vi "Read config file.vi"(3 "error in":errorcluster, 4 "file (use dialog)":path) -> (0 "error out":errorcluster, 1 "Drives":T2(array[cluster]))   [LabVIEW 2014]
uses:
  Axis enum.ctl
panel:
  out "Drive letters":string[](array[string])
  # "GUI=22\nAXES=2 CE\nC:XRT1=109\nE:XLA3=1250\nC:RANGE=360\nE:RANGE=50\nLEVEL=2\nCL=1"
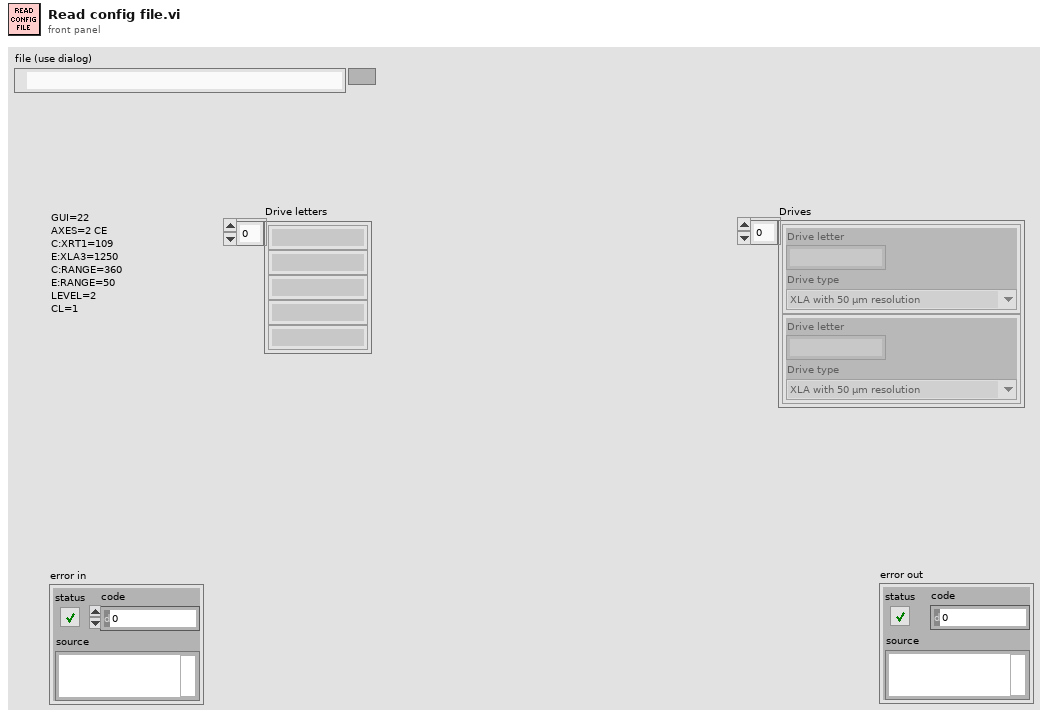
[diagram p1: front panel]
types:
  T1 = typedef "Axis enum.ctl" = enum16{"XLA with 50 µm resolution", "XLA with 10 µm resolution", "XLA with 1250 nm resolution", "XLA with 312 nm resolution", "XLA with 78 nm resolution", "XLS with 1250 nm resolution", "XLS with 312 nm resolution", "XLS with 78nm resolution", "XLS with 5nm resolution", "XLS with 1 nm resolution", "XRT-A with 109 µrad resolution", "XRT-U-30 with 109 µrad resolution", "XRT-U-30 with 49 µrad resolution", "XRT-U-30 with 19 µrad resolution", "XRT-U-30 with 3 µrad resolution", "XRT-U-40 with 109 µrad resolution", "XRT-U 40 with 49 µrad resolution", "XRT-U-40 with 19 µrad resolution", "XRT-U-40 with 3 µrad resolution", "XRT-U-60 with 109 µrad resolution", "XRT-U-60 with 49 µrad resolution", "XRT-U-60 with 19 µrad resolution", "XRT-U-60 with 3 µrad resolution"}
  T2 = cluster{"Drive letter":string, "Drive type":T1}[]
  T3 = cluster{"Name":string, "Data":string, "Enum type":T1}[]
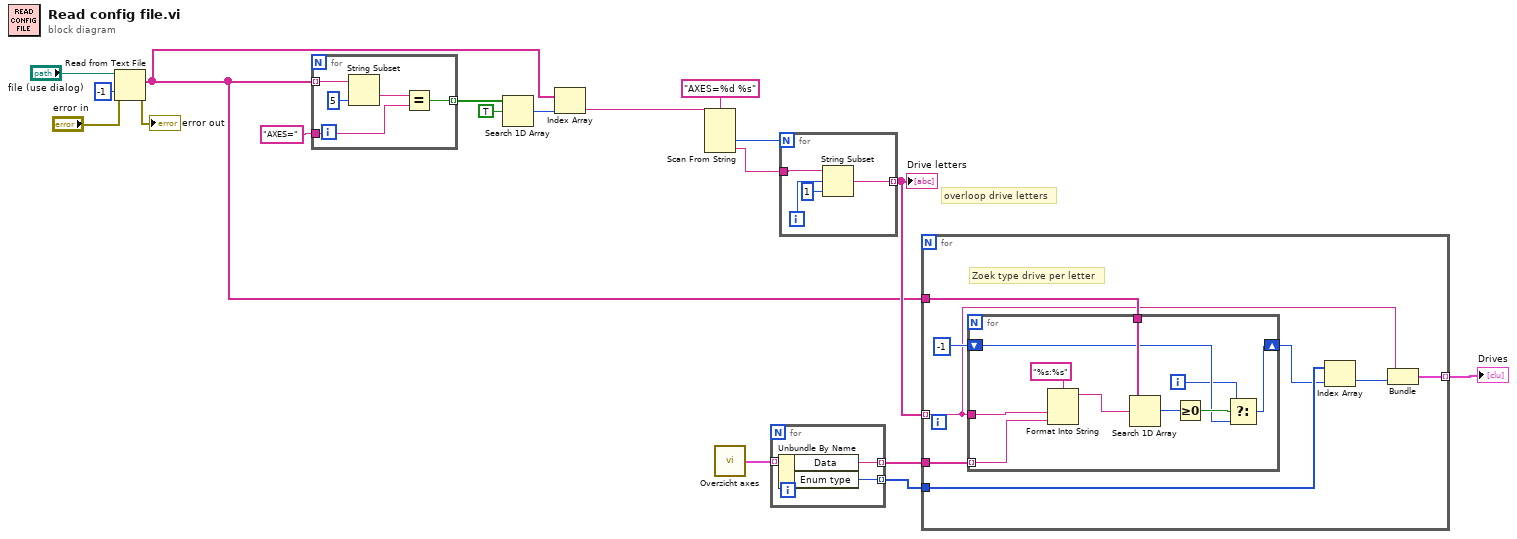
[diagram p0: block diagram]
diagram:
  # "overloop drive letters"
  n1 = Read from Text File(file (use dialog)="file (use dialog)", count=-1, error in="error in") -> (text=w2:string[], error out=→"error out":errorcluster)  [unwired: 1 in, 2 out]
  n2 = for {
    tunnel: w2 -> [w23] mode=indexing
    tunnel: [w20] -> w13 mode=indexing
    tunnel: "AXES=" ("y") -> [w19]
    n3 = String Subset(string=w23, length (rest)=5 ("length (rest)")) -> (substring=w21:string)  [unwired: 1 in]
    n4 = Equal?(x=w21, y=w19) -> (x = y?=w20:bool)
  }
  n5 = Search 1D Array(1D array=w13, element=TRUE) -> (index of element=w11:i32)  [unwired: 1 in]
  n6 = Index Array(array=w2, index=w11) -> (element=w9:string)
  n7 = Scan From String(format string="AXES=%d %s", input string=w9) -> (output 1=w7:i32, output 2=w6:string)  [unwired: 4 in, 3 out]
  n8 = call "Overzicht axes.vi"() -> ("Data out"=w15:T3)  [unwired: 5 in]
  n9 = for {
    tunnel: w15 -> [w26] mode=indexing
    tunnel: [w25] -> w5 mode=indexing
    tunnel: [w24] -> w4 mode=indexing
    n10 = Unbundle By Name(w26) -> ("Data"=w25:string, "Enum type"=w24:T1)
  }
  n11 = for {
    N: w7 -> [_]
    tunnel: w6 -> [w30]
    tunnel: [w27] -> w3 mode=indexing
    i -> [w29]
    n12 = String Subset(string=w30, offset (0)=w29, length (rest)=1 ("length (rest)")) -> (substring=w27:string)
  }
  "Drive letters" <- w3
  n13 = for {
    tunnel: w3 -> [w33] mode=indexing
    tunnel: w5 -> [w36]
    tunnel: w4 -> [w38]
    tunnel: w2 -> [w35]
    tunnel: [w32] -> w1 mode=indexing
    # "Zoek type drive per letter"
    n14 = for {
      tunnel: w33 -> [w48]
      tunnel: w36 -> [w46] mode=indexing
      tunnel: w35 -> [w44]
      shift-right: [w40] -> w31
      shift-left: -1 -> [w42]
      i -> [w39]
      n15 = Format Into String(format string="%s:%s", w48, w46) -> (resulting string=w45:string)  [unwired: 2 in, 1 out]
      n16 = Search 1D Array(1D array=w44, element=w45) -> (index of element=w41:i32)  [unwired: 1 in]
      n17 = Greater Or Equal To 0?(x=w41) -> (x >= 0?=w43:bool)
      n18 = Select(t=w39, s=w43, f=w42) -> (s? t:f=w40:i32)
    }
    n19 = Index Array(array=w38, index=w31) -> (element=w37:T1)
    n20 = Bundle(w33, "Enum type"=w37) -> (w32:cluster{string, "Enum type":T1})  [unwired: 1 in]
  }
  "Drives" <- w1
